vi "Init ABORT.vi"(8 "error in (no error)":errorcluster, 11 "Guardian in":refnum<class "Guardian.lvclass">) -> (0 "error out":errorcluster, 3 "Guardian out":refnum<class "Guardian.lvclass">)   [LabVIEW 2026, in "TALOS.lvlib" / "Guardian.lvlib" / "Guardian.lvclass"]
uses:
  Guardian.lvclass
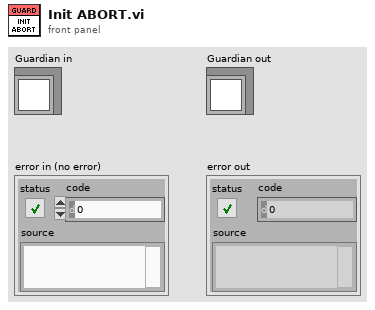
[diagram p1: front panel]
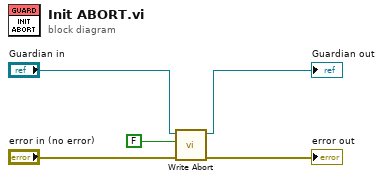
[diagram p0: block diagram]
diagram:
  n1 = call "Write Abort.vi"("error in (no error)"="error in (no error)", "Abort value"=FALSE ("Abort"), "Guardian in"="Guardian in") -> ("error out"=→"error out":errorcluster, "Guardian out"=→"Guardian out":refnum<class "Guardian.lvclass">)  [unwired: 7 in]
